vi "Read Gain.vi"(8 "error in (no error)":errorcluster, 11 "Cible in":refnum<class "Cible.lvclass">) -> (0 "error out":errorcluster, 2 "Gain":dbl, 3 "Cible out":refnum<class "Cible.lvclass">)   [LabVIEW 2017, in "Cible.lvclass"]
uses:
  Cible.lvclass
  Cible.lvclass/Cible.ctl
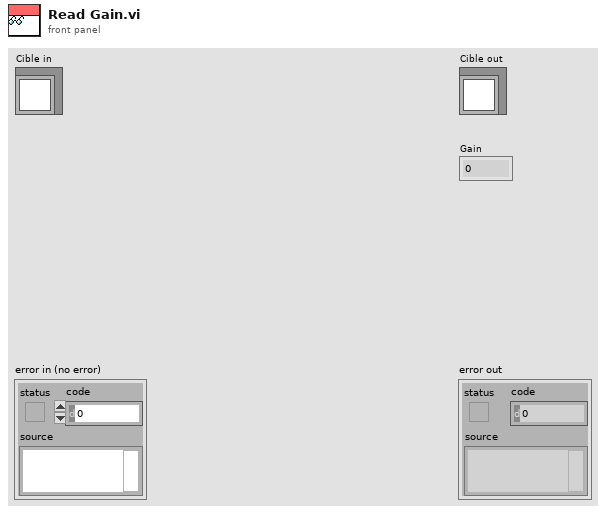
[diagram p1: front panel]
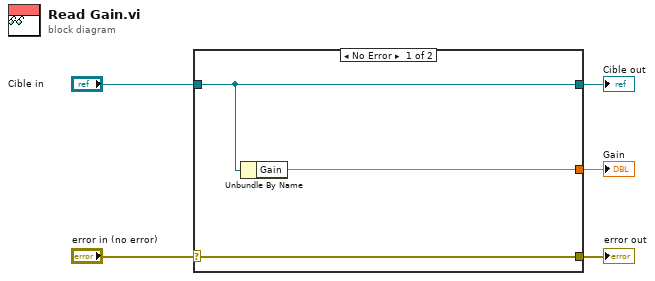
[diagram p0: block diagram]
diagram:
  n1 = case shown="No Error" "error in (no error)" {
    selector: "error in (no error)" -> [w8 w9]
    tunnel: [w8 w9] -> w4
    tunnel: [w7 w10] -> w2
    tunnel: "Cible in" -> [w7 w10]
    tunnel: [w6 _] -> w1
    frame No Error {
      n2 = Unbundle By Name(w7) -> ("Gain"=w6:dbl)
    }
    frame Error {
    }
  }
  "error out" <- w4
  "Cible out" <- w2
  "Gain" <- w1
